vi "VINameToVI.vi"(8 "error in (no error)":errorcluster, 10 "vi":string, 11 "Application in":refnum<vi>) -> (0 "error out":errorcluster, 3 "VI out":refnum<vi>)   [LabVIEW 2021]
uses:
  <vilib>/regexp/Match Regular Expression.xnode
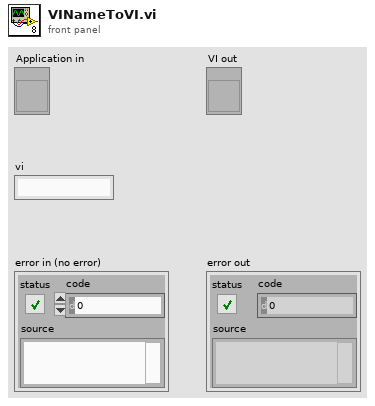
[diagram p1: front panel]
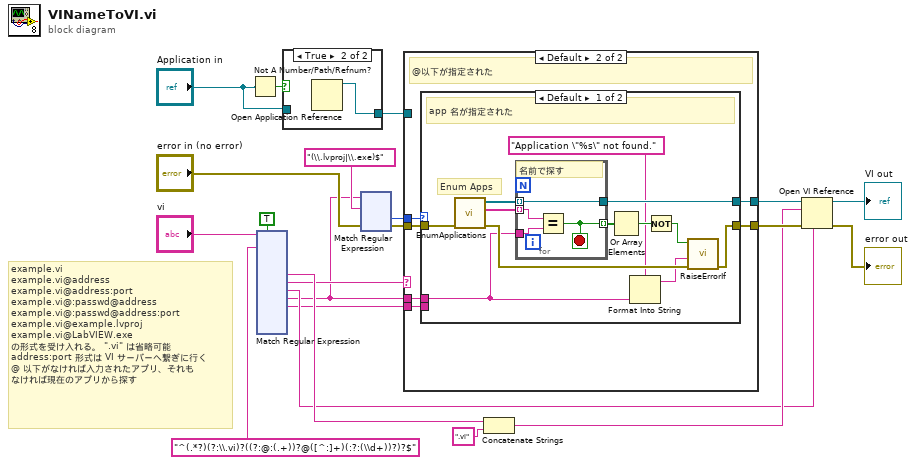
[diagram p0: block diagram]
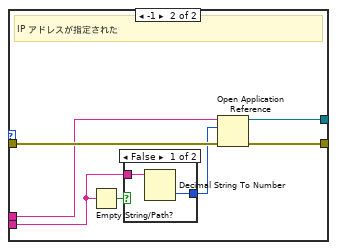
[diagram p4: hidden frame]
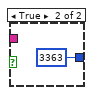
[diagram p5: hidden frame]
diagram:
  # "example.vi\nexample.vi@address\nexample.vi@address:port\nexample.vi@:passwd@address\nexample.vi@:passwd@address:port\nexample.vi@example.lvproj\nexample.vi@LabVIEW.exe\nの形式を受け入れる。 \".vi\" は省略可能\naddress:port 形式は VI サーバーへ繋ぎに行く\n@ 以下がなければ入力されたアプリ、それも\nなければ現在のアプリから探す"
  n1 = Not A Number/Path/Refnum?(number/path/refnum="Application in") -> (NaN/Path/Refnum?=w15:bool)
  n2 = xnode "Match Regular Expression"("input string"="vi", "regular expression"="^(.*?)(?:\\.vi)?((?:@:(.+))?@([^:]+)(:?:(\\d+))?)?$" ("input string"), "ignore case? (F)"=TRUE) -> ("submatch 1"=w17:string, "submatch 2"=w4:string, "submatch 3"=w3:string, "submatch 4"=w2:string, "submatch 5"=w1:string)  [unwired: 3 in, 8 out]
  n3 = case shown="True" w15 {
    tunnel: "Application in" -> [w22 _]
    tunnel: [w22 w23] -> w7
    frame False {
    }
    frame True {
      n4 = Open Application Reference() -> (3:w23:refnum<vi>)  [unwired: 4 in, 1 out]
    }
  }
  n5 = xnode "Match Regular Expression"("input string"=w2, "regular expression"="(\\.lvproj|\\.exe)$", "error in"="error in (no error)") -> ("offset past match"=w9:i32, "error out"=w5:errorcluster)  [unwired: 3 in, 3 out]
  n6 = case shown="Default" w4 {
    tunnel: w5 -> [w24 w31]
    tunnel: w2 -> [_ w30]
    tunnel: w1 -> [_ w29]
    tunnel: [w24 w28] -> w13
    tunnel: [w25 w27] -> w12
    tunnel: w9 -> [_ w26]
    tunnel: w7 -> [w25 _]
    frame "" {
    }
    frame Default {
      # "@以下が指定された"
      n7 = case shown="Default" w26 {
        tunnel: w31 -> [w43 w54]
        tunnel: w29 -> [_ w51]
        tunnel: w30 -> [w33 w50]
        tunnel: [w36 w48] -> w28
        tunnel: [w39 w49] -> w27
        frame Default {
          # "Enum Apps"
          # "app 名が指定された"
          n8 = call "EnumApplications.vi"("error in (no error)"=w43) -> ("error out"=w40:errorcluster, "Application Names"=w41:string[], "Application References"=w42:refnum<vi>[])  [unwired: 8 in]
          n9 = for {
            tunnel: w42 -> [w44] mode=indexing
            tunnel: w41 -> [w47] mode=indexing
            tunnel: w33 -> [w46]
            tunnel: [w45] -> w38 mode=indexing
            tunnel: [w44] -> w39
            stop <- w45 stop-if-true
            # "名前で探す"
            n10 = Equal?(x=w47, y=w46) -> (x = y?=w45:bool)
          }
          n11 = Or Array Elements(Boolean array=w38) -> (logical OR=w37:bool)
          n12 = Format Into String(format string="Application \"%s\" not found." ("error message"), w33) -> (resulting string=w32:string)  [unwired: 2 in, 1 out]
          n13 = Not(x=w37) -> (.not. x?=w35:bool)
          n14 = call "RaiseErrorIf.vi"("error in (no error)"=w40, "error message"=w32, "error? (true)"=w35) -> ("error out"=w36:errorcluster)  [unwired: 8 in]
        }
        frame -1 {
          # "IP アドレスが指定された"
          n15 = Empty String/Path?(string/path=w51) -> (empty?=w53:bool)
          n16 = case shown="False" w53 {
            tunnel: w51 -> [w56 _]
            tunnel: [w55 3363] -> w52
            frame False {
              n17 = Decimal String To Number(string=w56) -> (number=w55:i32)  [unwired: 2 in, 1 out]
            }
            frame True {
            }
          }
          n18 = Open Application Reference(8:w54, 10:w52, 11:w50) -> (0:w48:errorcluster, 3:w49:refnum<vi>)  [unwired: 1 in]
        }
      }
    }
  }
  n19 = Concatenate Strings(w17, ".vi" ("string")) -> (w8:string)
  n20 = Open VI Reference(application reference (local)=w12, vi path=w8, password ("")=w3, error in (no error)=w13) -> (vi reference=→"VI out":refnum<vi>, error out=→"error out":errorcluster)  [unwired: 2 in]
